vi "HexStr2NorStr.vi"(9 "Hex Display":string) -> (1 "Normal Display":string)   [LabVIEW 2017]
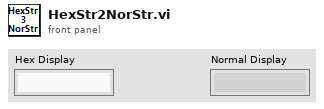
[diagram p1: front panel]
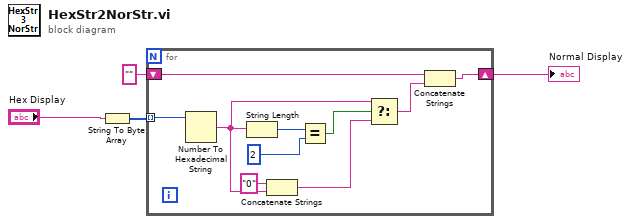
[diagram p0: block diagram]
diagram:
  n1 = String To Byte Array(string="Hex Display") -> (unsigned byte array=w1:u8[])
  n2 = for {
    shift-right: [w13] -> w4
    shift-left: "" -> [w14]
    tunnel: w1 -> [w12] mode=indexing
    n3 = Number To Hexadecimal String(2:w12) -> (0:w8:string)  [unwired: 1 in]
    n4 = String Length(string=w8) -> (length=w11:i32)
    n5 = Concatenate Strings("0" ("字符串"), w8) -> (w9:string)
    n6 = Equal?(x=w11, y=2) -> (x = y?=w5:bool)
    n7 = Select(t=w8, s=w5, f=w9) -> (s? t:f=w6:string)
    n8 = Concatenate Strings(w14, w6) -> (w13:string)
  }
  "Normal Display" <- w4
